vi "平行样流程汇总.vi"(11 "参数":T1) -> ()   [LabVIEW 2016, in "质控单元.lvlib"]
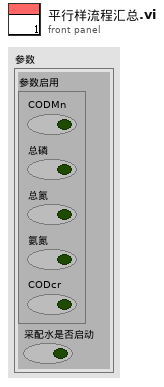
[diagram p1: front panel]
types:
  T1 = cluster{"参数启用":cluster{"CODMn":bool, "总磷":bool, "总氮":bool, "氨氮":bool, "CODcr":bool}, "采配水是否启动":bool}
  T2 = enum32{"Bad", "Idle", "Run top level", "Running"}
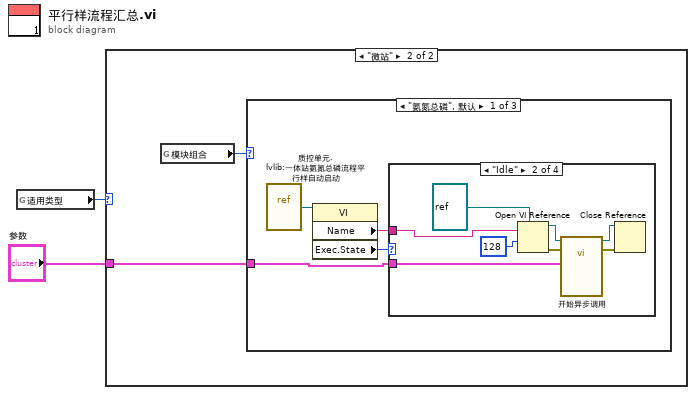
[diagram p0: block diagram]
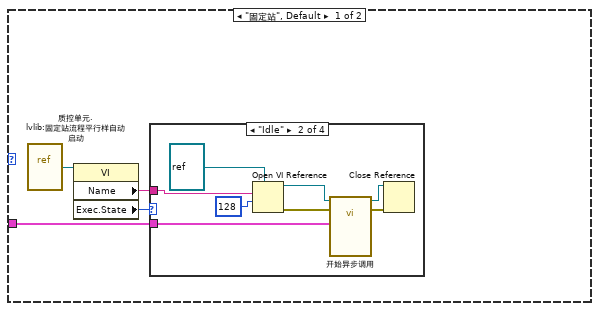
[diagram p2: hidden frame]
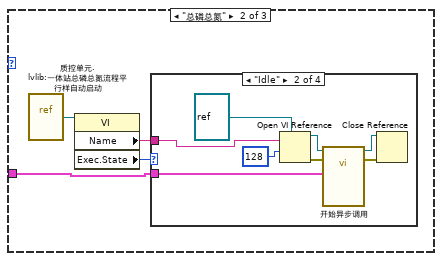
[diagram p9: hidden frame]
diagram:
  n1 = global read "断电保存全局.vi" "适用类型"() -> (w2:enum16{"固定站", "微站"})
  n2 = case shown="\"微站\"" w2 {
    tunnel: "参数" -> [w3 w15]
    frame "固定站", Default {
      n3 = vi-ref "质控单元.lvlib:固定站流程平行样自动启动.vi"() -> (w5:refnum<vi>)
      n4 = property class="VI"(reference=w5) -> ("Name"=w6:string, "Exec.State"=w4:T2)  [unwired: 1 in, 2 out]
      n5 = case shown="\"Idle\"" w4 {
        tunnel: w6 -> [_ w13 _ _]
        tunnel: w3 -> [_ w7 _ _]
        frame "Bad", Default {
        }
        frame "Idle" {
          n6 = Open VI Reference(type specifier VI Refnum (for type only)=refnum<vi> refnum ("类型说明符VI引用句柄（仅用于类型）"), vi path=w13, options=128 ("选项")) -> (vi reference=w14:refnum<vi>, error out=w10:errorcluster)  [unwired: 3 in]
          n7 = call-by-ref "开始异步调用"(reference=w14, error in=w10, "参数"=w7) -> (reference out=w12:refnum<vi>, error out=w11:errorcluster)  [unwired: 11 in]
          n8 = Close Reference(reference=w12, error in (no error)=w11) -> ()  [unwired: 1 out]
        }
        frame "Run top level" {
        }
        frame "Running" {
        }
      }
    }
    frame "微站" {
      n9 = global read "断电保存全局.vi" "模块组合"() -> (w16:enum16{"氨氮总磷", "总磷总氮", "氨氮、总磷、总氮"})
      n10 = case shown="\"氨氮总磷\", 默认" w16 {
        tunnel: w15 -> [w17 w29 _]
        frame "氨氮总磷", Default {
          n11 = vi-ref "质控单元.lvlib:一体站氨氮总磷流程平行样自动启动.vi"() -> (w19:refnum<vi>)
          n12 = property class="VI"(reference=w19) -> ("Name"=w20:string, "Exec.State"=w18:T2)  [unwired: 1 in, 2 out]
          n13 = case shown="\"Idle\"" w18 {
            tunnel: w20 -> [_ w27 _ _]
            tunnel: w17 -> [_ w21 _ _]
            frame "Bad", Default {
            }
            frame "Idle" {
              n14 = Open VI Reference(type specifier VI Refnum (for type only)=refnum<vi> refnum ("类型说明符VI引用句柄（仅用于类型）"), vi path=w27, options=128 ("选项")) -> (vi reference=w28:refnum<vi>, error out=w24:errorcluster)  [unwired: 3 in]
              n15 = call-by-ref "开始异步调用"(reference=w28, error in=w24, "参数"=w21) -> (reference out=w26:refnum<vi>, error out=w25:errorcluster)  [unwired: 11 in]
              n16 = Close Reference(reference=w26, error in (no error)=w25) -> ()  [unwired: 1 out]
            }
            frame "Run top level" {
            }
            frame "Running" {
            }
          }
        }
        frame "总磷总氮" {
          n17 = vi-ref "质控单元.lvlib:一体站总磷总氮流程平行样自动启动.vi"() -> (w31:refnum<vi>)
          n18 = property class="VI"(reference=w31) -> ("Name"=w32:string, "Exec.State"=w30:T2)  [unwired: 1 in, 2 out]
          n19 = case shown="\"Idle\"" w30 {
            tunnel: w32 -> [_ w39 _ _]
            tunnel: w29 -> [_ w33 _ _]
            frame "Bad", Default {
            }
            frame "Idle" {
              n20 = Open VI Reference(type specifier VI Refnum (for type only)=refnum<vi> refnum ("类型说明符VI引用句柄（仅用于类型）"), vi path=w39, options=128 ("选项")) -> (vi reference=w40:refnum<vi>, error out=w36:errorcluster)  [unwired: 3 in]
              n21 = call-by-ref "开始异步调用"(reference=w40, error in=w36, "参数"=w33) -> (reference out=w38:refnum<vi>, error out=w37:errorcluster)  [unwired: 11 in]
              n22 = Close Reference(reference=w38, error in (no error)=w37) -> ()  [unwired: 1 out]
            }
            frame "Run top level" {
            }
            frame "Running" {
            }
          }
        }
        frame "氨氮、总磷、总氮" {
        }
      }
    }
  }
